vi "格式化取.vi"() -> ()   [LabVIEW 2018]
panel:
  out "输出 3":dbl
  out "输出 2":bool
  out "输出 1":string
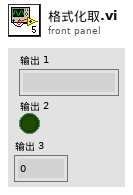
[diagram p1: front panel]
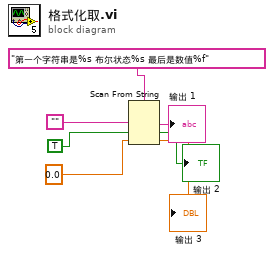
[diagram p0: block diagram]
diagram:
  n1 = Scan From String("第一个字符串是%s 布尔状态%s 最后是数值%f" ("格式字符串"), default 1="", default 2=TRUE, default 3=0.0) -> (output 1=→"输出 1":string, output 2=→"输出 2":bool, output 3=→"输出 3":dbl)  [unwired: 2 in, 2 out]
